vi "Set_Coords.vi"(8 "function name":string="read_translation_from_file", 9 "Filepath":string="C:\\Users\\conno.DESKTOP-98EBONR\\OneDrive\\Desktop\\GitHub Repo\\Ko_Group_Software_Apps\\Python Codes\\STM Automation Codes\\latest_translation_flat.txt", 10 "module path":path=path "C:/Users/conno.DESKTOP-98EBONR/OneDrive/Desktop/GitHub Repo/Ko_Group_Software_Apps/Python Codes/STM Automation Codes/Python_LV_Tran_Commo.py", 11 "Python version":string="3.9") -> (2 "return value":cluster{"x":dbl, "y":dbl}, 3 "Filepath  2":string)   [LabVIEW 2025]
panel:
  in  "Cluster":cluster{"x":dbl, "y":dbl}
  out "error out":errorcluster
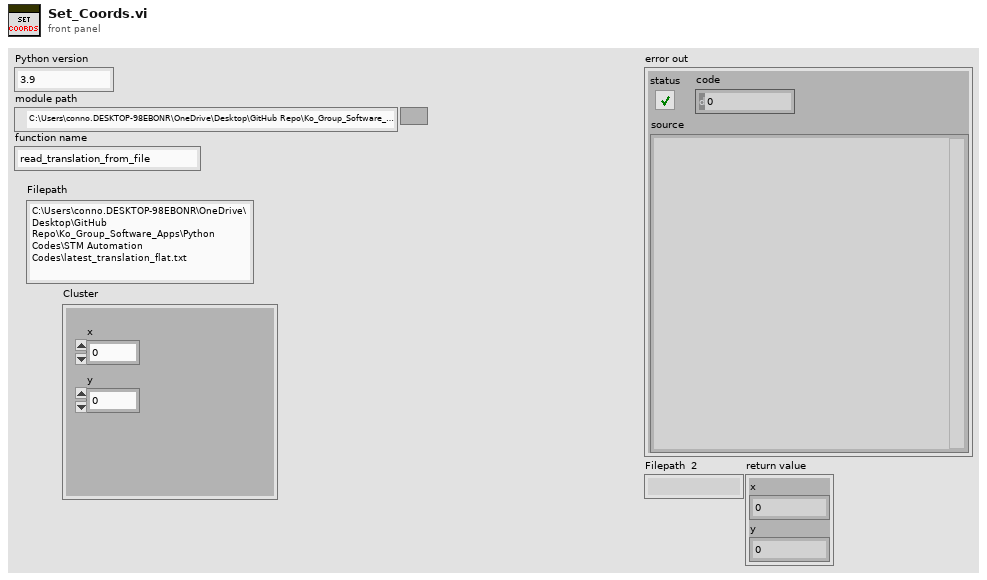
[diagram p1: front panel]
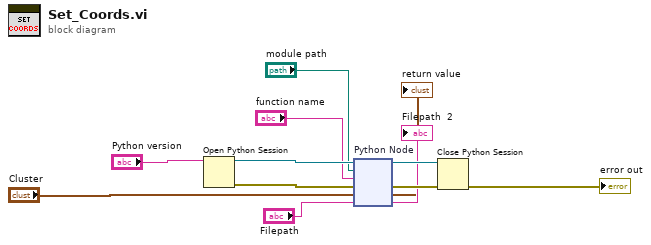
[diagram p0: block diagram]
diagram:
  n1 = Open Python Session(python version="Python version") -> (session out=w12:refnum<k35>, error out=w11:errorcluster)  [unwired: 2 in]
  n2 = node "Python Node"(w12, "module path", "function name", w11, "Cluster", "Filepath") -> (w9:refnum<k35>, w10:errorcluster, →"return value":cluster{"x":dbl, "y":dbl}, →"Filepath  2":string)  [unwired: 2 out]
  n3 = Close Python Session(session in=w9, error in=w10) -> (11:→"error out":errorcluster)
